vi "Remove missing Waveforms.vi"(7 "Names to Remove":string[](array[string]), 8 "Error In":errorcluster, 9 "ListBox Variant In":variant, 10 "CD Settings in":T2 {"CD Task Dependency Ref" format="%.0x"; "CD Task Dependency" format="%.0x"}, 11 "Item Ref In":T1 format="%.0x") -> (0 "Error Out":errorcluster, 1 "ListBox Variant Out":variant, 2 "CD Settings out":T2 {"CD Task Dependency Ref" format="%.0x"; "CD Task Dependency" format="%.0x"}, 3 "Item Ref Out":T1 format="%.0x")   [LabVIEW 2017, in "Waveform-Processing-Custom-Device System Explorer.lvlib"]
doc: "This application is provided the list of \"Selected Waveforms\" and the channels to be removed. this is required because the Analog Input channel was renamed and must be removed from the output array so that it can be re-added as desired."
uses:
  Waveform-Processing-Custom-Device System Explorer.lvlib
  Shared/Custom Device Settings.ctl
  <vilib>/NI Veristand/Custom Device API/Custom Device Item Ref.ctl
  <vilib>/NI Veristand/Custom Device Tools/Custom Device Utility Library/NI VeriStand - Search for Item by Name.vi
  <vilib>/NI VeriStand/Custom Device API/Custom Device API.lvlib
  <vilib>/NI VeriStand/Custom Device Tools/Custom Device Utility Library/Custom Device Utility Library.lvlib
  Shared/Waveform-Processing-Custom-Device Shared.lvlib
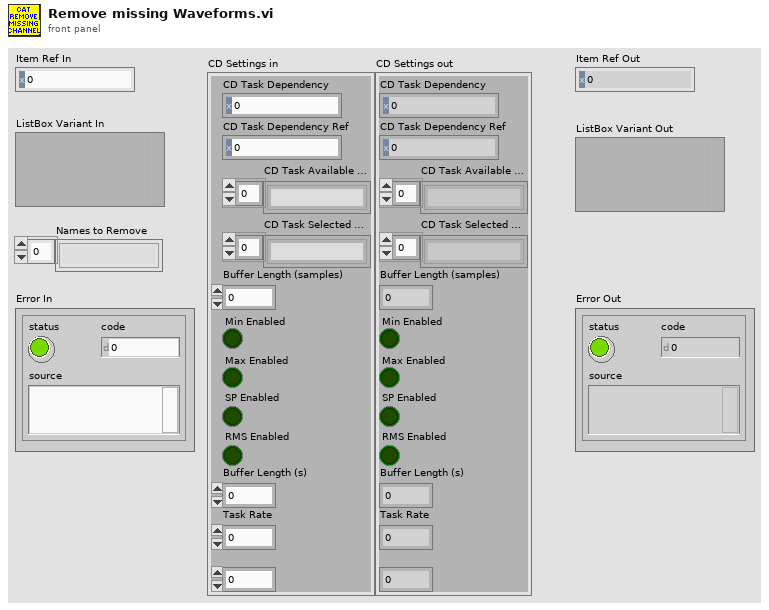
[diagram p1: front panel]
types:
  T1 = typedef "Custom Device API.lvlib/Custom Device Item Ref.ctl" = u64
  T2 = typedef "Waveform-Processing-Custom-Device Shared.lvlib/Custom Device Settings.ctl" = cluster{"CD Task Dependency":T1, "CD Task Dependency Ref":T1, "CD Task Available Wfms":string[], "CD Task Selected Wfms":string[], "Buffer Length (samples)":u32, "Min Enabled":bool, "Max Enabled ":bool, "SP Enabled":bool, "RMS Enabled":bool, "Buffer Length (s)":dbl, "Task Rate":dbl, "Number of DAQ Chanels":u32}
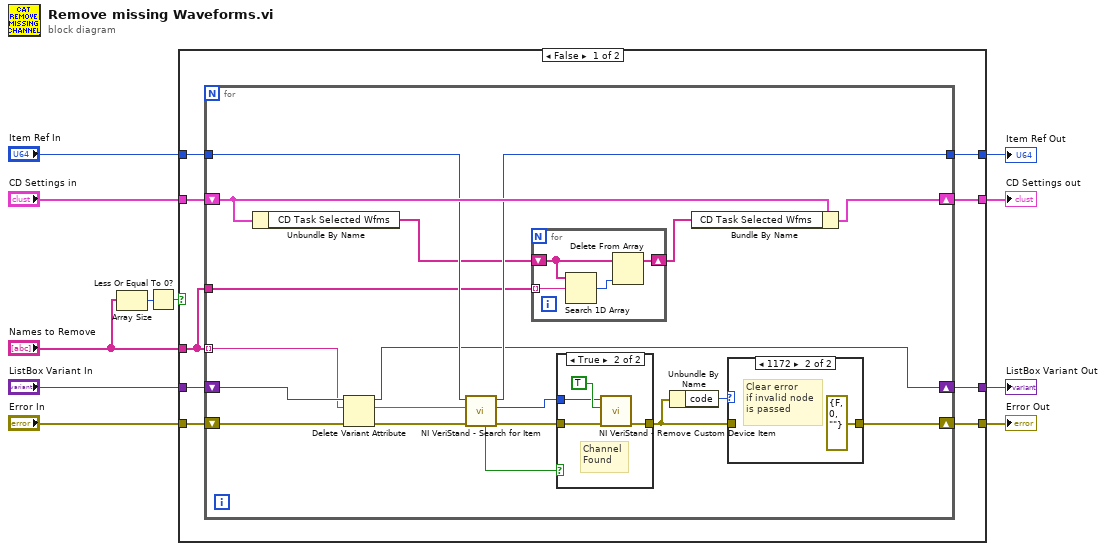
[diagram p0: block diagram]
diagram:
  n1 = Array Size(array="Names to Remove") -> (size(s)=w3:i32)
  n2 = Less Or Equal To 0?(x=w3) -> (x <= 0?=w2:bool)
  n3 = case shown="False" w2 {
    tunnel: [w20 w52] -> w11
    tunnel: "CD Settings in" -> [w19 w52]
    tunnel: "Item Ref In" -> [w18 w53]
    tunnel: [w17 w53] -> w8
    tunnel: [w16 w50] -> w7
    tunnel: "ListBox Variant In" -> [w15 w51]
    tunnel: "Error In" -> [w14 w50]
    tunnel: [w13 w51] -> w4
    tunnel: "Names to Remove" -> [w12 _]
    frame False {
      n4 = for {
        tunnel: w12 -> [w25] mode=indexing
        shift-right: [w27] -> w13
        shift-left: w15 -> [w29]
        shift-right: [w22] -> w16
        shift-left: w14 -> [w28]
        tunnel: w18 -> [w33]
        tunnel: [w32] -> w17
        tunnel: w12 -> [w23]
        shift-right: [w38] -> w20
        shift-left: w19 -> [w37]
        n5 = Unbundle By Name(w37) -> ("CD Task Selected Wfms"=w24:string[])
        n6 = Delete Variant Attribute(4:w28, 6:w25, 7:w29) -> (0:w26:errorcluster, 3:w27:variant)  [unwired: 1 out]
        n7 = call-poly <vilib>:"NI VeriStand - Search for Item.vi"("error in"=w26, "Item Name"=w25, "Section Ref in"=w33) -> ("error out"=w34:errorcluster, "Item Ref"=w35:T1, "Section Ref out"=w32:T1, "Found"=w36:bool)  [unwired: 5 in]
        n8 = for {
          shift-right: [w42] -> w21
          shift-left: w24 -> [w40]
          tunnel: w23 -> [w39] mode=indexing
          n9 = Search 1D Array(1D array=w40, element=w39) -> (index of element=w41:i32)  [unwired: 1 in]
          n10 = Delete From Array(array=w40, index=w41) -> (array with subset deleted=w42:string[])  [unwired: 1 in, 1 out]
        }
        n11 = case shown="True" w36 {
          tunnel: [w45 w48] -> w30
          tunnel: w34 -> [w45 w47]
          tunnel: w35 -> [_ w46]
          frame False {
            # "Channel\n   NOT \nFound"
          }
          frame True {
            # "Channel\nFound"
            n12 = call <vilib>:"NI VeriStand - Remove Custom Device Item.vi"("error in (no error)"=w47, "Force Delete (F)"=TRUE, "Item Ref in"=w46) -> ("error out"=w48:errorcluster)  [unwired: 7 in, 1 out]
          }
        }
        n13 = Unbundle By Name(w30) -> ("code"=w31:i32)
        n14 = Bundle By Name(cluster=w37, "CD Task Selected Wfms"=w21) -> (w38:T2)
        n15 = case shown="1172" w31 {
          tunnel: w30 -> [w43 _]
          tunnel: [w43 errorcluster {"status"=FALSE, "code"=0, "source"=""} ("error out")] -> w22
          frame 0, Default {
          }
          frame 1172 {
            # "Clear error\nif invalid node\nis passed"
          }
        }
      }
    }
    frame True {
    }
  }
  "ListBox Variant Out" <- w4
  "CD Settings out" <- w11
  "Item Ref Out" <- w8
  "Error Out" <- w7
